vi "PV ActiveLine - Gas Type Correction (TPG362).vi"(7 "W/R":bool, 8 "Fehler (Eingang)":errorcluster, 9 "Gas S 2":i8(ring) items=["no channel"=-1, "Nitrogen"=0, "Argon"=1, "Hydrogen"=2, "Helium"=3, "Neon"=4, "Krypton"=5, "Xenon"=6, "other"=7], 10 "Gas S 1":i8(ring) items=["Nitrogen", "Argon", "Hydrogen", "Helium", "Neon", "Krypton", "Xenon", "other"], 11 "Referenz in":refnum<visa-resource-name>) -> (0 "Cluster (Ausgang)":errorcluster, 1 "Gas Out 2":i8(ring) items=["Nitrogen", "Argon", "Hydrogen", "Helium", "Neon", "Krypton", "Xenon", "other"], 2 "Gas Out 1":i8(ring) items=["Nitrogen", "Argon", "Hydrogen", "Helium", "Neon", "Krypton", "Xenon", "other"], 3 "Referenz out":refnum<visa-resource-name>)   [LabVIEW 2013, in "PV ActiveLine.lvlib"]
doc: "GAS – Gas Type Correction\n\nTransmit: GAS [a,a]\nReceive: a,a\n\nGas type correction,\na =\n0 –> nitrogen / air (default)\n1 –> Argon\n2 –> Hydrogen\n3 –> Helium\n4 –> Neon\n5 –> Krypton\n6 –> Xenon\n7 –> Other gases"
uses:
  <instrlib>/PV ActiveLine/PV ActiveLine.lvlib
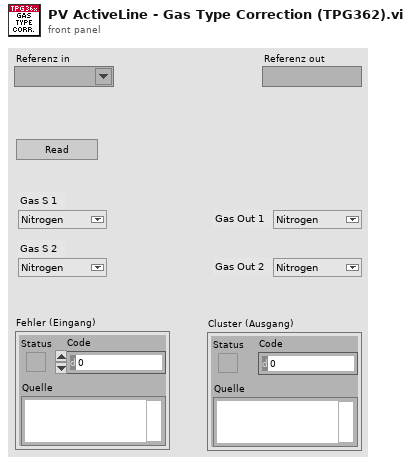
[diagram p1: front panel]
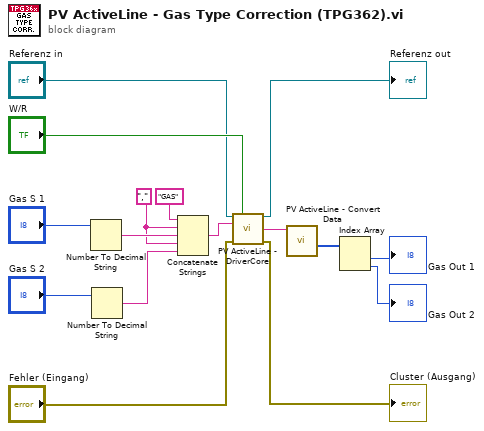
[diagram p0: block diagram]
diagram:
  w2 = ","
  n1 = Number To Decimal String(number="Gas S 1") -> (decimal integer string=w3:string)  [unwired: 1 in]
  n2 = Number To Decimal String(number="Gas S 2") -> (decimal integer string=w1:string)  [unwired: 1 in]
  n3 = Concatenate Strings("GAS", w2, w3, w2, w1) -> (w10:string)
  n4 = call <instrlib>:"PV ActiveLine - DriverCore.vi"("Referenz in"="Referenz in", "Write/Read"="W/R", "Command"=w10, "Fehler (Eingang)"="Fehler (Eingang)") -> ("Referenz out"=→"Referenz out":refnum<visa-resource-name>, "String Out"=w7:string, "Cluster (Ausgang)"=→"Cluster (Ausgang)":errorcluster)  [unwired: 9 in]
  n5 = call <instrlib>:"PV ActiveLine - Convert Data.vi"("String in"=w7) -> ("Integer Out"=w6:i32[])  [unwired: 7 in, 3 out]
  n6 = Index Array(array=w6) -> (element #1=→"Gas Out 1":i32, element #2=→"Gas Out 2":i32)  [unwired: 2 in]
